vi "Flatten.vi"(8 "error in (no error)":errorcluster, 11 "LCD Reader in":refnum<class "LCD Reader.lvclass">) -> (0 "error out":errorcluster, 3 "LCD Reader out":refnum<class "LCD Reader.lvclass">)   [LabVIEW 2023, in "LCD Reader.lvclass"]
uses:
  LCD Reader.lvclass
  LCD Reader.lvclass/LCD Reader.ctl
  Global/File Locations.vi
  Reader/Reader.lvclass
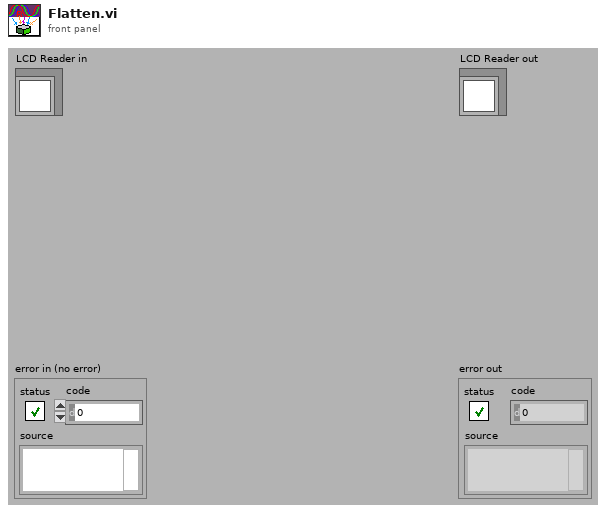
[diagram p1: front panel]
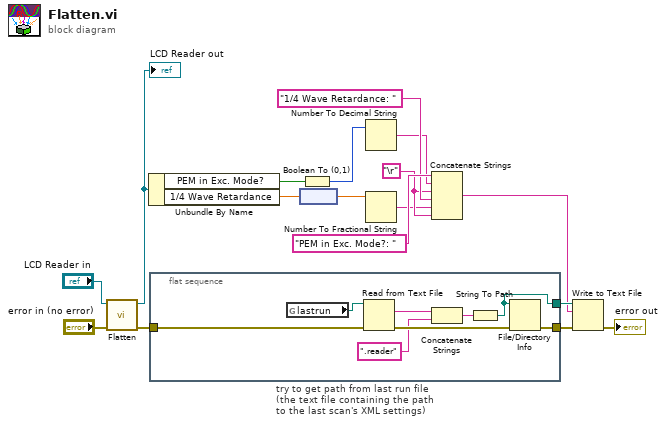
[diagram p0: block diagram]
diagram:
  w4 = "\r"
  n1 = call-parent "Flatten.vi"("error in (no error)"="error in (no error)", "Reader in"="LCD Reader in") -> ("error out"=w15:errorcluster, "Reader out"=w11:refnum<class "LCD Reader.lvclass">)  [unwired: 8 in]
  "LCD Reader out" <- w11
  n2 = Unbundle By Name(w11) -> ("PEM in Exc. Mode?"=w10:bool, "1/4 Wave Retardance"=w8:dbl[unit])
  n3 = flat-sequence "try to get path from last run file\n(the text file containing the path\nto the last scan's XML settings)" {
    tunnel: [w25] -> w12
    tunnel: [w22] -> w13
    tunnel: w15 -> [w21]
    frame #0 {
      n4 = global read "File Locations.vi" "lastrun"() -> (w24:path)
      n5 = Read from Text File(file (use dialog)=w24, error in=w21) -> (text=w20:string, error out=w23:errorcluster)  [unwired: 4 out]
      n6 = Concatenate Strings(w20, ".reader") -> (w18:string)
      n7 = String To Path(string=w18) -> (path=w25:path)
      n8 = File/Directory Info(path=w25, error in=w23) -> (error out=w22:errorcluster)  [unwired: 6 out]
    }
  }
  n9 = node(w8) -> (w7:dbl)
  n10 = Boolean To (0,1)(Boolean=w10) -> (0, 1=w9:i16)
  n11 = Number To Decimal String(number=w9) -> (decimal integer string=w3:string)  [unwired: 1 in]
  n12 = Number To Fractional String(number=w7) -> (F-format string=w2:string)  [unwired: 3 in]
  n13 = Concatenate Strings("PEM in Exc. Mode?: ", w3, w4, "1/4 Wave Retardance: ", w2, w4) -> (w1:string)
  n14 = Write to Text File(file (use dialog)=w12, text=w1, error in=w13) -> (error out=→"error out":errorcluster)  [unwired: 1 in, 2 out]
